vi "StdM.vi"(11 "2D in":dbl[][](array[numeric])) -> (0 "1D Std":dbl[](array[numeric]), 1 "[Xi-X]":dbl[][](array[numeric]), 2 "Xi - X":dbl[](array[numeric]), 3 "Mean":dbl[](array[numeric]) format="%#_4g", 4 "Mean from first row":dbl format="%#_4g")   [LabVIEW 2023]
uses:
  <vilib>/Analysis/NI_AALBase.lvlib
panel:
  out "size(s)":i32[](array[numeric])
  out "variance":dbl[](array[numeric]) format="%#_4g"
  out "My Variance":dbl[](array[numeric]) format="%#_4g"
  out "std":dbl[](array[numeric])
  out "mean":dbl[](array[numeric]) format="%#_4g"
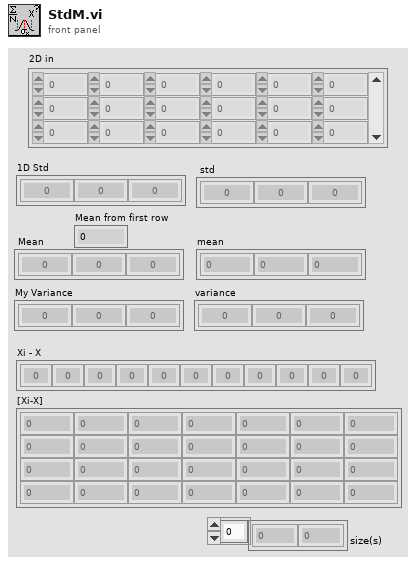
[diagram p1: front panel]
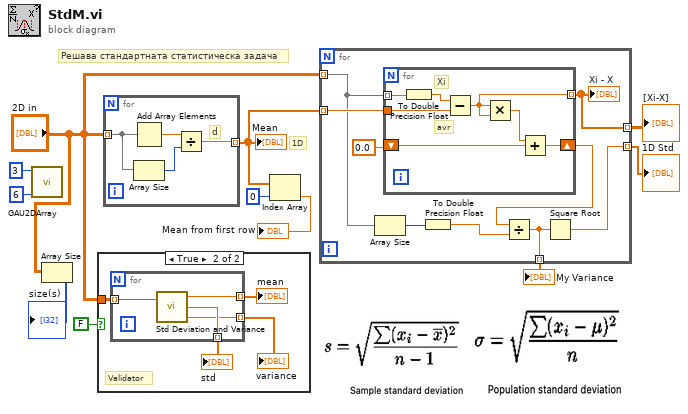
[diagram p0: block diagram]
diagram:
  # "1D"
  # "Решава стандартната статистическа задача"
  n1 = call "GAU2DArray.vi"("Colums"=6, "Rows"=3) -> ()  [unwired: 7 in, 3 out]
  n2 = Array Size(array="2D in") -> (size(s)=→"size(s)":i32[])
  n3 = case shown="True" FALSE {
    tunnel: "2D in" -> [_ w13]
    frame False {
    }
    frame True {
      # "Validator"
      n4 = for {
        tunnel: w13 -> [w19] mode=indexing
        tunnel: [w18] -> w15 mode=indexing
        tunnel: [w17] -> w14 mode=indexing
        tunnel: [w16] -> w12 mode=indexing
        n5 = call <vilib>:"Std Deviation and Variance.vi"("X"=w19) -> ("mean"=w18:dbl, "standard deviation"=w17:dbl, "variance"=w16:dbl)  [unwired: 1 in]
      }
      "mean" <- w15
      "std" <- w14
      "variance" <- w12
    }
  }
  n6 = for {
    tunnel: "2D in" -> [w21] mode=indexing
    tunnel: [w20] -> w5 mode=indexing
    # "d"
    n7 = Add Array Elements(numeric array=w21) -> (sum=w23:dbl)
    n8 = Array Size(array=w21) -> (size(s)=w22:i32)
    n9 = Divide(x=w23, y=w22) -> (x/y=w20:dbl)
  }
  "Mean" <- w5
  n10 = Index Array(array=w5, index=0) -> (element=→"Mean from first row":dbl)
  n11 = for {
    tunnel: "2D in" -> [w30] mode=indexing
    tunnel: w5 -> [w32] mode=indexing
    tunnel: [w28] -> w9 mode=indexing
    tunnel: [w26] -> w8 mode=indexing
    tunnel: [w25] -> w6 mode=indexing
    n12 = Array Size(array=w30) -> (size(s)=w29:i32)
    n13 = for {
      tunnel: w30 -> [w38] mode=indexing
      tunnel: w32 -> [w39]
      shift-right: [w34] -> w27
      shift-left: 0.0 -> [w35]
      tunnel: [w33] -> w25 mode=indexing
      # "Xi"
      # "avr"
      n14 = To Double Precision Float(number=w38) -> (double precision float=w37:dbl)
      n15 = Subtract(x=w37, y=w39) -> (x-y=w33:dbl)
      n16 = Multiply(x=w33, y=w33) -> (x*y=w36:dbl)
      n17 = Add(x=w36, y=w35) -> (x+y=w34:dbl)
    }
    "Xi - X" <- w25
    n18 = To Double Precision Float(number=w29) -> (double precision float=w24:dbl)
    n19 = Divide(x=w27, y=w24) -> (x/y=w26:dbl)
    n20 = Square Root(x=w26) -> (sqrt(x)=w28:dbl)
  }
  "1D Std" <- w9
  "My Variance" <- w8
  "[Xi-X]" <- w6
